vi "xijk_load_from_file.vi"(8 "error in":errorcluster, 11 "file path (dialog if empty)":path) -> (0 "error out":errorcluster, 3 "load cluster out":T1={{"axes in"={"min x-axis excitation"=0, "max x-axis excitation"=0, "min x-axis emission"=0, "max x-axis emission"=0, "precision of results"=2}, "plot colors in"={"Lanscape Portrait"=FALSE, "Plot logarithmic"=FALSE, "Ex/Em filters double"=FALSE, "Line colors"=[]}}, "search paths in"={"Paths"={"Path: Excitation filters"=path "", "Path: Dicroic filters"=path "", "Path: Emission filters"=path "", "Path reget"=path ""}, "table excitation"=[], "table dicroics"=[], "table emission"=[], "Integers"={"Select result number"=0}, "boolean selector array"=[], "table for calculation automagic"=[]}, "spectra parameters in"={"Booleans"={"Unknown detector"=FALSE, "Dual band filters"=FALSE, "Dual emission by cubes"=FALSE, "FRET"=FALSE}, "Integers"={"Light source"=0, "Number of fluorophores"=0, "Wavelength of laser (nm) 1"=0, "Broadness of laser (nm) 1"=0.0, "Wavelength of laser (nm) 2"=0, "Broadness of laser (nm) 2"=0.0, "Template"=0}, "Doubles"={"Molar extinction 1"=0.0, "Molar extinction 2"=0.0, "Quantum efficiency 1"=0.0, "Quantum efficiency 2"=0.0}}, "filepaths in"={"Excitation filter 1"=path "", "Dichroic filter 1"=path "", "Emission filter 1"=path "", "Excitation filter 2"=path "", "Dichroic filter 2"=path "", "Emission filter 2"=path "", "Extra em filter 1"=path "", "Extra em filter 2"=path "", "Light source file"=path "", "Fluorophore absorption 1"=path "", "Fluorophore emission 1"=path "", "Fluorophore absorption 2"=path "", "Fluorophore emission 2"=path "", "Detector"=path ""}} {"?"."axes in"."precision of results" max=8 step=1})   [LabVIEW 2009]
uses:
  Type Def/save_cluster.ctl
  Type Def/configuration_cluster.ctl
  Type Def/axis_parameters.ctl
  Type Def/color_parameters.ctl
  Type Def/search_parameters.ctl
  Type Def/spectra_parameters.ctl
  Type Def/filepath.ctl
  <vilib>/Utility/xml.llb/Read From XML File(array).vi
panel:
  in  "load cluster in":T1={{"axes in"={"min x-axis excitation"=0, "max x-axis excitation"=0, "min x-axis emission"=0, "max x-axis emission"=0, "precision of results"=2}, "plot colors in"={"Lanscape Portrait"=FALSE, "Plot logarithmic"=FALSE, "Ex/Em filters double"=FALSE, "Line colors"=[]}}, "search paths in"={"Paths"={"Path: Excitation filters"=path "", "Path: Dicroic filters"=path "", "Path: Emission filters"=path "", "Path reget"=path ""}, "table excitation"=[], "table dicroics"=[], "table emission"=[], "Integers"={"Select result number"=0}, "boolean selector array"=[], "table for calculation automagic"=[]}, "spectra parameters in"={"Booleans"={"Unknown detector"=FALSE, "Dual band filters"=FALSE, "Dual emission by cubes"=FALSE, "FRET"=FALSE}, "Integers"={"Light source"=0, "Number of fluorophores"=0, "Wavelength of laser (nm) 1"=0, "Broadness of laser (nm) 1"=0.0, "Wavelength of laser (nm) 2"=0, "Broadness of laser (nm) 2"=0.0, "Template"=0}, "Doubles"={"Molar extinction 1"=0.0, "Molar extinction 2"=0.0, "Quantum efficiency 1"=0.0, "Quantum efficiency 2"=0.0}}, "filepaths in"={"Excitation filter 1"=path "", "Dichroic filter 1"=path "", "Emission filter 1"=path "", "Excitation filter 2"=path "", "Dichroic filter 2"=path "", "Emission filter 2"=path "", "Extra em filter 1"=path "", "Extra em filter 2"=path "", "Light source file"=path "", "Fluorophore absorption 1"=path "", "Fluorophore emission 1"=path "", "Fluorophore absorption 2"=path "", "Fluorophore emission 2"=path "", "Detector"=path ""}} {"?"."axes in"."precision of results" max=8 step=1}
  # "Dichroic"
  # "Ex/Em filter"
  # "Fluorophore 1"
  # "Fluorophore 2"
  # "Laser /\nextra Em filter"
  # "Dichroic"
  # "Ex/Em filter"
  # "Fluorophore 1"
  # "Fluorophore 2"
  # "Laser /\nextra Em filter"
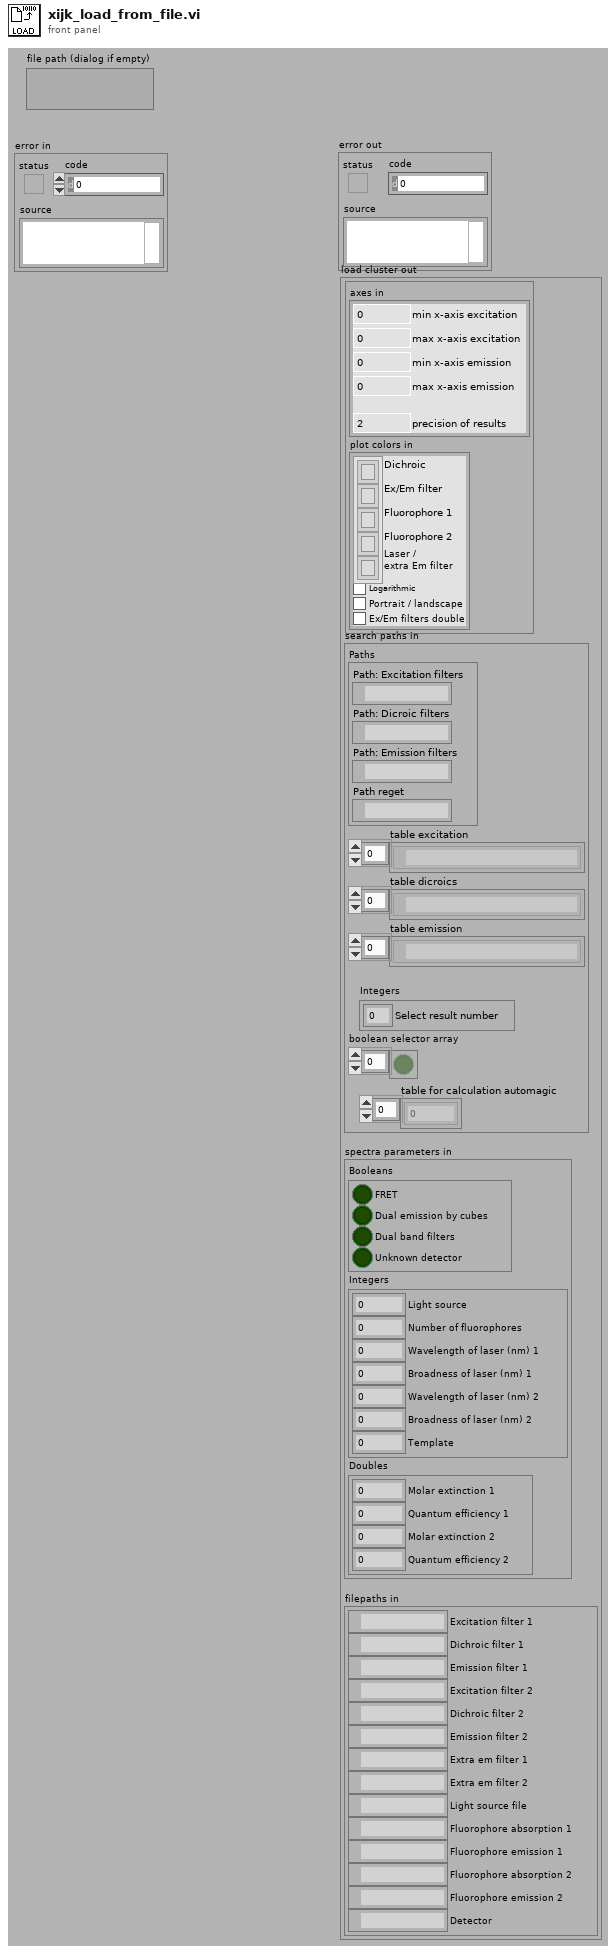
[diagram p1: front panel]
types:
  T1 = typedef "save_cluster.ctl" = cluster{T2, "search paths in":T5, "spectra parameters in":T6, "filepaths in":T7}
  T2 = typedef "configuration_cluster.ctl" = cluster{"axes in":T3, "plot colors in":T4}
  T3 = typedef "axis_parameters.ctl" = cluster{"min x-axis excitation":u16, "max x-axis excitation":u16, "min x-axis emission":u16, "max x-axis emission":u16, "precision of results":u8}
  T4 = typedef "color_parameters.ctl" = cluster{"Lanscape Portrait":bool, "Plot logarithmic":bool, "Ex/Em filters double":bool, "Line colors":u32[]}
  T5 = typedef "search_parameters.ctl" = cluster{"Paths":cluster{"Path: Excitation filters":path, "Path: Dicroic filters":path, "Path: Emission filters":path, "Path reget":path}, "table excitation":path[], "table dicroics":path[], "table emission":path[], "Integers":cluster{"Select result number":u32}, "boolean selector array":bool[], "table for calculation automagic":i32[]}
  T6 = typedef "spectra_parameters.ctl" = cluster{"Booleans":cluster{"Unknown detector":bool, "Dual band filters":bool, "Dual emission by cubes":bool, "FRET":bool}, "Integers":cluster{"Light source":u16, "Number of fluorophores":u16, "Wavelength of laser (nm) 1":u16, "Broadness of laser (nm) 1":sgl, "Wavelength of laser (nm) 2":u16, "Broadness of laser (nm) 2":sgl, "Template":u16}, "Doubles":cluster{"Molar extinction 1":sgl, "Molar extinction 2":sgl, "Quantum efficiency 1":sgl, "Quantum efficiency 2":sgl}}
  T7 = typedef "filepath.ctl" = cluster{"Excitation filter 1":path, "Dichroic filter 1":path, "Emission filter 1":path, "Excitation filter 2":path, "Dichroic filter 2":path, "Emission filter 2":path, "Extra em filter 1":path, "Extra em filter 2":path, "Light source file":path, "Fluorophore absorption 1":path, "Fluorophore emission 1":path, "Fluorophore absorption 2":path, "Fluorophore emission 2":path, "Detector":path}
  T8 = cluster{"[0]":path, "[1]":path, "[2]":path, "[3]":path, "[4]":path, "[5]":path, "[6]":path, "[7]":path, "[8]":path, "[9]":path, "[10]":path, "[11]":path, "[12]":path, "[13]":path}
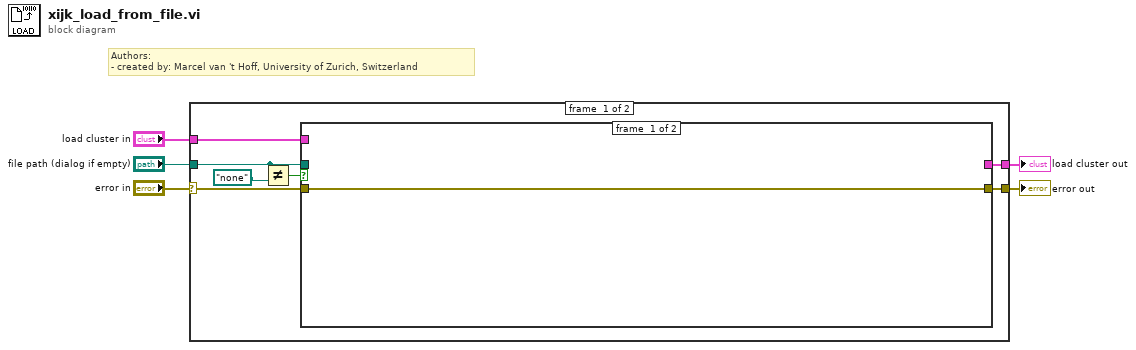
[diagram p0: block diagram]
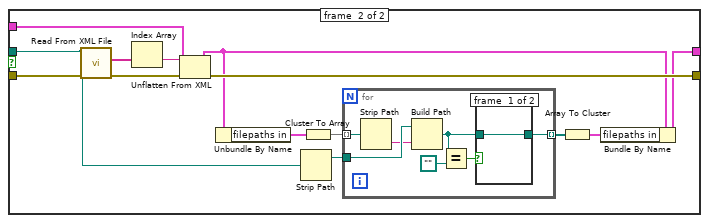
[diagram p2: hidden frame]
diagram:
  # "Authors: \n- created by: Marcel van 't Hoff, University of Zurich, Switzerland"
  n1 = case shown="No Error" "error in" {
    selector: "error in" -> [w12 w36]
    tunnel: [w11 w36] -> w4
    tunnel: "file path (dialog if empty)" -> [w6 _]
    tunnel: "load cluster in" -> [w10 _]
    tunnel: [w9 _] -> w1
    frame #0 {
      n2 = Not Equal?(x=w6, y=path "none") -> (x != y?=w8:bool)
      n3 = case shown="True" w8 {
        tunnel: w6 -> [_ w20]
        tunnel: w12 -> [w13 w26]
        tunnel: [w13 w23] -> w11
        tunnel: w10 -> [_ w22]
        tunnel: [_ w14] -> w9
        frame #0 {
        }
        frame #1 {
          n4 = call-poly <vilib>:"Read From XML File.vi"("error in (no error)"=w26, "XML File Path"=w20) -> ("error out"=w24:errorcluster, "XML Elements"=w27:string[])  [unwired: 7 in, 1 out]
          n5 = Index Array(array=w27) -> (element=w25:string)  [unwired: 1 in]
          n6 = Unflatten From XML(xml string=w25, type=w22, error in (no error)=w24) -> (value=w15:T1, error out=w23:errorcluster)
          n7 = Unbundle By Name(w15) -> ("filepaths in"=w17:T7)
          n8 = Strip Path(path=w20) -> (stripped path=w19:path)  [unwired: 1 out]
          n9 = Cluster To Array(cluster=w17) -> (array=w21:path[])
          n10 = for {
            tunnel: w21 -> [w34] mode=indexing
            tunnel: w19 -> [w33]
            tunnel: [w28] -> w18 mode=indexing
            n11 = Strip Path(path=w34) -> (name=w32:string)  [unwired: 1 out]
            n12 = Build Path(base path=w33, name or relative path=w32) -> (appended path=w29:path)
            n13 = Equal?(x=w29, y=path "") -> (x = y?=w30:bool)
            n14 = case shown="True" w30 {
              tunnel: w29 -> [w35 _]
              tunnel: [w35 _] -> w28
              frame #0 {
              }
              frame #1 {
              }
            }
          }
          n15 = Array To Cluster(array=w18) -> (cluster=w16:T8)
          n16 = Bundle By Name(cluster=w15, "filepaths in"=w16) -> (w14:T1)
        }
      }
    }
    frame #1 {
    }
  }
  "error out" <- w4
  "load cluster out" <- w1
